vi "Move Tree Items Under Parents.vi"(8 "error in":errorcluster, 11 "state in":T1) -> (0 "error out":errorcluster, 3 "state out":T1)   [LabVIEW 2010, in "NI_SE_Config Front Panel Layout.lvlib"]
uses:
  NI_SE_Config Front Panel Layout.lvlib
  State.ctl
  VI Info.ctl
  VI Panel Layout/VI Panel Layout.lvclass
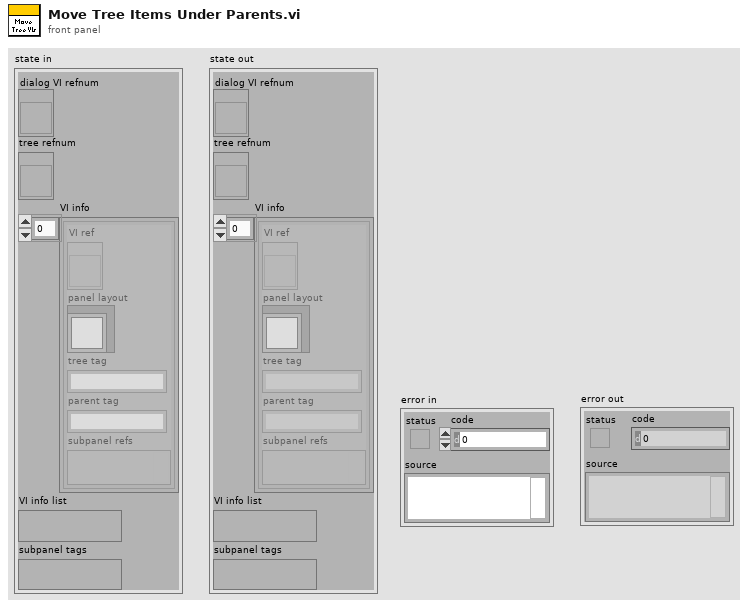
[diagram p1: front panel]
types:
  T1 = typedef "NI_SE_Config Front Panel Layout.lvlib/State.ctl" = cluster{"dialog VI refnum":refnum<vi>, "tree refnum":refnum<vi>, "VI info":T2[], "VI info list":variant, "subpanel tags":variant}
  T2 = typedef "NI_SE_Config Front Panel Layout.lvlib/VI Info.ctl" = cluster{"VI ref":refnum<vi>, "panel layout":refnum<class "VI Panel Layout.lvclass">, "tree tag":string, "parent tag":string, "subpanel refs":variant}
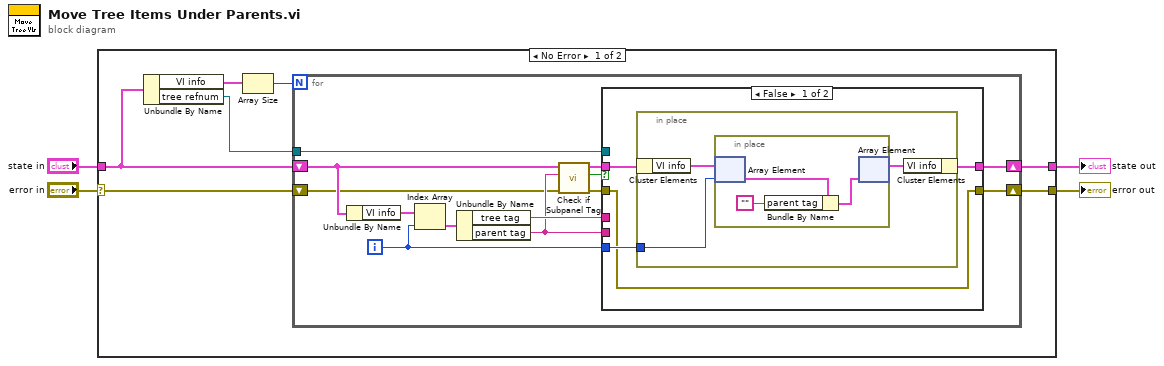
[diagram p0: block diagram]
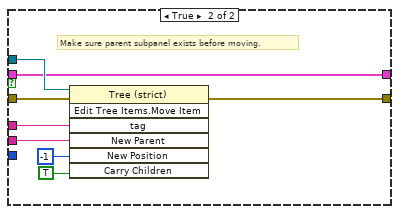
[diagram p2: hidden frame]
diagram:
  n1 = case shown="No Error" "error in" {
    selector: "error in" -> [w10 w43]
    tunnel: "state in" -> [w5 w44]
    tunnel: [w6 w44] -> w2
    tunnel: [w11 w43] -> w1
    frame No Error {
      n2 = Unbundle By Name(w5) -> ("VI info"=w9:T2[], "tree refnum"=w7:refnum<vi>)
      n3 = Array Size(array=w9) -> (size(s)=w8:i32)
      n4 = for {
        N: w8 -> [_]
        shift-right: [w19] -> w11
        shift-left: w10 -> [w13]
        shift-right: [w20] -> w6
        shift-left: w5 -> [w15]
        tunnel: w7 -> [w21]
        i -> [w18]
        n5 = Unbundle By Name(w15) -> ("VI info"=w23:T2[])
        n6 = Index Array(array=w23, index=w18) -> (element=w24:T2)
        n7 = Unbundle By Name(w24) -> ("tree tag"=w22:string, "parent tag"=w14:string)
        n8 = call "Check if Subpanel Tag.vi"("error in"=w13, "subpanel tag"=w14, "state in"=w15) -> ("error out"=w12:errorcluster, "found?"=w17:bool, "state out"=w16:T1)  [unwired: 4 in, 2 out]
        n9 = case shown="False" w17 {
          tunnel: w12 -> [w25 w38]
          tunnel: w22 -> [_ w40]
          tunnel: w14 -> [_ w39]
          tunnel: w21 -> [_ w37]
          tunnel: w16 -> [w28 w36]
          tunnel: [w27 w36] -> w20
          tunnel: [w25 w35] -> w19
          tunnel: w18 -> [w26 _]
          frame False {
            n10 = in-place {
              in-place-border: w26 -> [w29]
              n11 = in-place-cluster #1(w28) -> ("VI info"=w31:T2[])
              n12 = in-place {
                n13 = in-place-array #2(w31, w29) -> (w34:T2)
                n14 = Bundle By Name(cluster=w34, "parent tag"="") -> (w33:T2)
                n15 = in-place-array #2(w33) -> (w30:T2[])  [unwired: 1 out]
              }
              n16 = in-place-cluster #1("VI info"=w30) -> (w27:T1)
            }
          }
          frame True {
            # "Make sure parent subpanel exists before moving."
            n17 = invoke class="Tree (strict)" method="Edit Tree Items.Move Item"(reference=w37, error in=w38, "tag"=w40, "New Parent"=w39, "New Position"=-1, "Carry Children"=TRUE ("Carry Children?")) -> (error out=w35:errorcluster)  [unwired: 1 in, 6 out]
          }
        }
      }
    }
    frame Error {
    }
  }
  "state out" <- w2
  "error out" <- w1
